vi "clLabview_BDPW_calc.vi"(0 "vi_lib.lvlib:clLabview.lvclass":refnum<class "clLabview.lvclass">, 2 "new Password":string="LVSR") -> (14 "MD5 password":string, 15 "Hash 1":string, 16 "Hash 2":string, 17 "MD5 password (Hex)":string, 18 "Hash 1 (Hex)":string, 19 "Hash 2 (Hex)":string)   [LabVIEW 2011, in "vi_lib.lvlib" / "clLabview.lvclass"]
uses:
  clLabview.lvclass
  clLabview.lvclass/clLabview.ctl
  vi_lib.lvlib
  clFileReader/clFileReader.lvclass
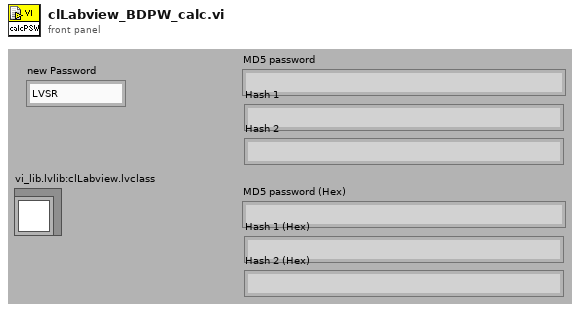
[diagram p1: front panel]
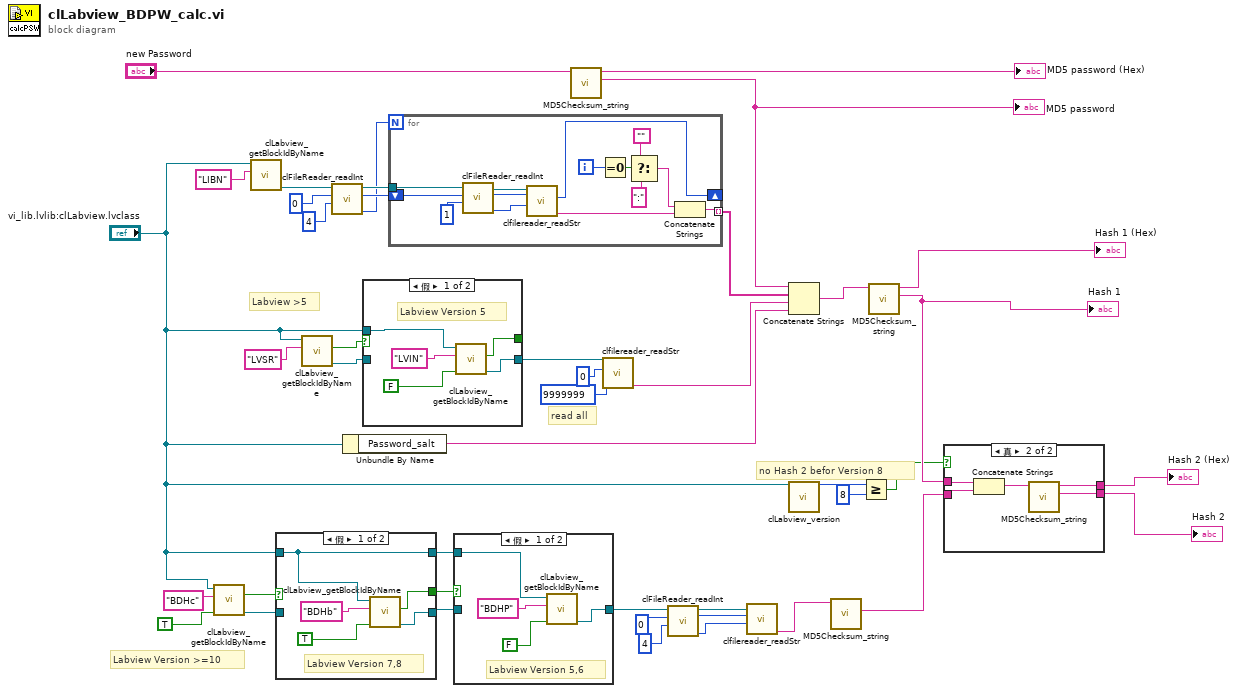
[diagram p0: block diagram]
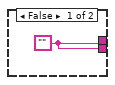
[diagram p2: hidden frame]
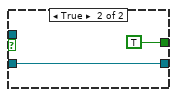
[diagram p3: hidden frame]
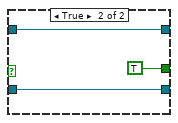
[diagram p5: hidden frame]
diagram:
  # "no Hash 2 befor Version 8"
  # "read all"
  # "Labview >5"
  # "Labview Version >=10"
  n1 = call "clLabview_getBlockIdByName.vi"("use compression (off)"=TRUE, "Block Name"="BDHc", "vi_lib.lvlib:clLabview.lvclass"="vi_lib.lvlib:clLabview.lvclass") -> ("Block Content"=w30:refnum<class "clFileReader.lvclass">, "Name found?"=w32:bool)  [unwired: 1 in, 5 out]
  n2 = call "clLabview_getBlockIdByName.vi"("Block Name"="LIBN", "vi_lib.lvlib:clLabview.lvclass"="vi_lib.lvlib:clLabview.lvclass") -> ("Block Content"=w39:refnum<class "clFileReader.lvclass">)  [unwired: 2 in, 6 out]
  n3 = case shown="假" w32 {
    tunnel: "vi_lib.lvlib:clLabview.lvclass" -> [w44 w49]
    tunnel: w30 -> [_ w51]
    tunnel: [w47 w51] -> w15
    tunnel: [w45 TRUE ("Name found?")] -> w14
    tunnel: [w44 w49] -> w6
    frame False {
      # "Labview Version 7,8"
      n4 = call "clLabview_getBlockIdByName.vi"("use compression (off)"=TRUE, "Block Name"="BDHb", "vi_lib.lvlib:clLabview.lvclass"=w44) -> ("Block Content"=w47:refnum<class "clFileReader.lvclass">, "Name found?"=w45:bool)  [unwired: 1 in, 5 out]
    }
    frame True {
    }
  }
  n5 = call "clLabview_getBlockIdByName.vi"("Block Name"="LVSR", "vi_lib.lvlib:clLabview.lvclass"="vi_lib.lvlib:clLabview.lvclass") -> ("Block Content"=w11:refnum<class "clFileReader.lvclass">, "Name found?"=w13:bool)  [unwired: 2 in, 5 out]
  n6 = call "clFileReader_readInt.vi"("size"=u32 4, "offset"=u32 0, "clFileReader.lvclass IN"=w39) -> ("OUT Value"=w7:u32, "new offset"=w9:u32, "clFileReader.lvclass OUT"=w10:refnum<class "clFileReader.lvclass">)  [unwired: 6 out]
  n7 = Unbundle By Name("vi_lib.lvlib:clLabview.lvclass") -> ("Password_salt"=w17:string)
  n8 = case shown="假" w13 {
    tunnel: "vi_lib.lvlib:clLabview.lvclass" -> [w56 _]
    tunnel: w11 -> [_ w58]
    tunnel: [w54 w58] -> w12
    tunnel: [w52 TRUE ("Name found?")] -> _
    frame False {
      # "Labview Version 5"
      n9 = call "clLabview_getBlockIdByName.vi"("use compression (off)"=FALSE, "Block Name"="LVIN", "vi_lib.lvlib:clLabview.lvclass"=w56) -> ("Block Content"=w54:refnum<class "clFileReader.lvclass">, "Name found?"=w52:bool)  [unwired: 1 in, 5 out]
    }
    frame True {
    }
  }
  n10 = for {
    N: w7 -> [_]
    tunnel: w10 -> [w72]
    tunnel: [w66] -> w8 mode=indexing
    shift-right: [w59] -> _
    shift-left: w9 -> [w60]
    i -> [w65]
    n11 = call "clFileReader_readInt.vi"("size"=u32 1, "offset"=w60, "clFileReader.lvclass IN"=w72) -> ("OUT Value"=w68:u32, "new offset"=w69:u32, "clFileReader.lvclass OUT"=w70:refnum<class "clFileReader.lvclass">)  [unwired: 6 out]
    n12 = call "clfilereader_readStr.vi"("size"=w68, "offset"=w69, "clFileReader.lvclass IN"=w70) -> ("ReadStr - OUT Value"=w67:string, "new offset"=w59:u32)  [unwired: 7 out]
    n13 = Equal To 0?(x=w65) -> (x = 0?=w64:bool)
    n14 = Select(t="", s=w64, f=":" ("ReadStr - OUT Value")) -> (s? t:f=w63:string)
    n15 = Concatenate Strings(w63, w67) -> (w66:string)
  }
  n16 = case shown="假" w14 {
    tunnel: w15 -> [_ w77]
    tunnel: [w75 w77] -> w16
    tunnel: w6 -> [w73 _]
    frame False {
      # "Labview Version 5,6"
      n17 = call "clLabview_getBlockIdByName.vi"("use compression (off)"=FALSE, "Block Name"="BDHP", "vi_lib.lvlib:clLabview.lvclass"=w73) -> ("Block Content"=w75:refnum<class "clFileReader.lvclass">)  [unwired: 1 in, 6 out]
    }
    frame True {
    }
  }
  n18 = call "MD5Checksum_string.vi"("Message String"="new Password") -> ("MD5 message-digest (Ascii)"=w19:string, "MD5 message-digest (Hex)"=→"MD5 password (Hex)":string)  [unwired: 9 out]
  "MD5 password" <- w19
  n19 = call "clfilereader_readStr.vi"("size"=u32 9999999, "offset"=u32 0, "clFileReader.lvclass IN"=w12) -> ("ReadStr - OUT Value"=w1:string)  [unwired: 8 out]
  n20 = call "clFileReader_readInt.vi"("size"=u32 4, "offset"=u32 0, "clFileReader.lvclass IN"=w16) -> ("OUT Value"=w24:u32, "new offset"=w25:u32, "clFileReader.lvclass OUT"=w26:refnum<class "clFileReader.lvclass">)  [unwired: 6 out]
  n21 = call "clfilereader_readStr.vi"("size"=w24, "offset"=w25, "clFileReader.lvclass IN"=w26) -> ("ReadStr - OUT Value"=w23:string)  [unwired: 8 out]
  n22 = Concatenate Strings(w19, w8, w1, w17) -> (w34:string)
  n23 = call "clLabview_version.vi"("vi_lib.lvlib:clLabview.lvclass"="vi_lib.lvlib:clLabview.lvclass") -> ("major"=w4:u8)  [unwired: 18 out]
  n24 = call "MD5Checksum_string.vi"("Message String"=w23) -> ("MD5 message-digest (Ascii)"=w21:string)  [unwired: 10 out]
  n25 = Greater Or Equal?(x=w4, y=u8 8) -> (x >= y?=w2:bool)
  n26 = call "MD5Checksum_string.vi"("Message String"=w34) -> ("MD5 message-digest (Ascii)"=w20:string, "MD5 message-digest (Hex)"=→"Hash 1 (Hex)":string)  [unwired: 9 out]
  "Hash 1" <- w20
  n27 = case shown="真" w2 {
    tunnel: [w78 w83] -> w22
    tunnel: w21 -> [_ w82]
    tunnel: w20 -> [_ w80]
    tunnel: [w78 w79] -> w18
    frame False {
      w78 = "" ("MD5 message-digest (Hex)")
    }
    frame True {
      n28 = Concatenate Strings(w80, w82) -> (w81:string)
      n29 = call "MD5Checksum_string.vi"("Message String"=w81) -> ("MD5 message-digest (Ascii)"=w79:string, "MD5 message-digest (Hex)"=w83:string)  [unwired: 9 out]
    }
  }
  "Hash 2 (Hex)" <- w22
  "Hash 2" <- w18
